vi "TEXT to Array.vi"(7 "My File has Row Headers":bool, 9 "precision (6)":i16, 11 "Spreadsheet path (.csv)":path=path "C:/Users/husmith/Desktop/MyData.csv") -> (2 "Data Dsiplay":dbl[][](array[numeric]), 3 "Spread Sheet Display":string[][](array[string]))   [LabVIEW 2015]
uses:
  <vilib>/Utility/file.llb/Read Delimited Spreadsheet (string).vi
  <vilib>/Utility/file.llb/Read Delimited Spreadsheet (DBL).vi
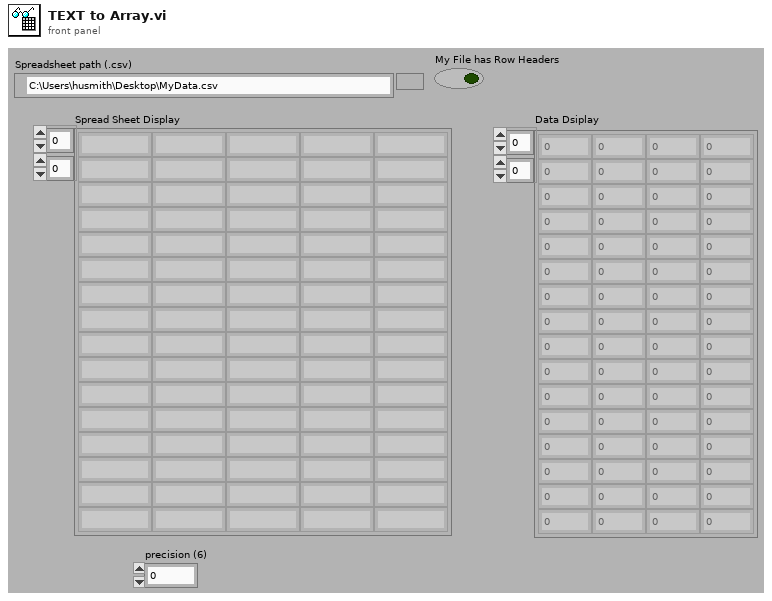
[diagram p1: front panel]
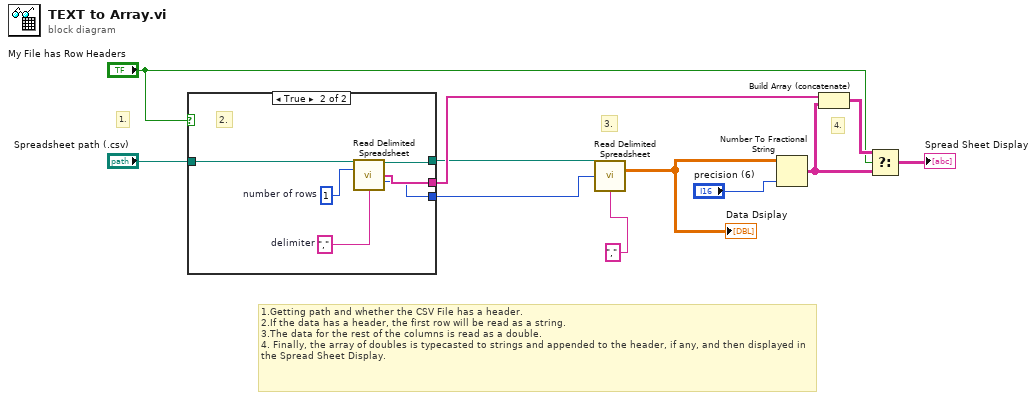
[diagram p0: block diagram]
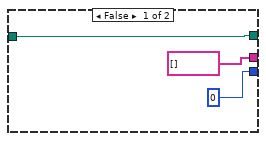
[diagram p2: hidden frame]
diagram:
  # "4."
  # "1.Getting path and whether the CSV File has a header.\n2.If the data has a header, the first row will be read as a string.\n3.The data for the rest of the columns is read as a double.\n4. Finally, the array of doubles is typecasted to strings and appended to the header, if any, and then displayed in the Spread Sheet Display."
  # "3."
  # "1."
  n1 = case shown="True" "My File has Row Headers" {
    tunnel: "Spreadsheet path (.csv)" -> [w12 w19]
    tunnel: [string[] [] ("first row") w17] -> w10
    tunnel: [0 ("mark after read (chars.)") w16] -> w2
    tunnel: [w12 w18] -> w3
    frame False {
    }
    frame True {
      w20 = 1  # number of rows
      w15 = ","  # delimiter
      # "2."
      n2 = call-poly <vilib>:"Read Delimited Spreadsheet.vi"("file path (dialog if empty)"=w19, "number of rows (all:-1)"=w20, "delimiter (\\t)"=w15) -> ("new file path (Not A Path if cancelled)"=w18:path, "first row"=w17:string[], "mark after read (chars.)"=w16:i32)  [unwired: 7 in, 3 out]
    }
  }
  n3 = call-poly <vilib>:"Read Delimited Spreadsheet.vi"("file path (dialog if empty)"=w3, "start of read offset (chars.:0)"=w2, "delimiter (\\t)"="," ("delimiter (\\t)")) -> ("all rows"=w1:dbl[][])  [unwired: 7 in, 5 out]
  "Data Dsiplay" <- w1
  n4 = Number To Fractional String(number=w1, precision (6)="precision (6)") -> (F-format string=w6:string[][])  [unwired: 2 in]
  n5 = Build Array (concatenate)(w10, w6) -> (w9:string[][])
  n6 = Select(t=w9, s="My File has Row Headers", f=w6) -> (s? t:f=→"Spread Sheet Display":string[][])
